vi "Create Folders.vi"(8 "error in (no error)":errorcluster, 11 "PostBuildSupport in":refnum<class "PostBuildSupport.lvclass">) -> (0 "error out":errorcluster, 3 "PostBuildSupport out":refnum<class "PostBuildSupport.lvclass">)   [LabVIEW 2016, in "PostBuildSupport.lvclass"]
uses:
  PostBuildSupport.lvclass
  PostBuildSupport.lvclass/PostBuildSupport.ctl
  <userlib>/_MGI/File/MGI Create Directory Chain Behavior Enum.ctl
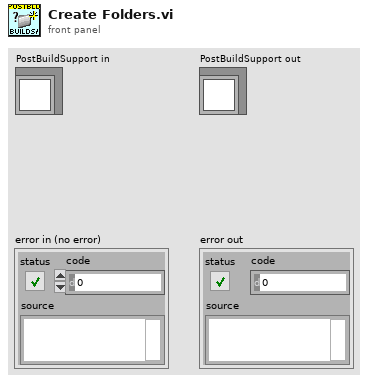
[diagram p1: front panel]
types:
  T1 = typedef "MGI Create Directory Chain Behavior Enum.ctl" = enum16{"Auto Detect", "Path Contains a File", "Path Does Not Contain a File"}
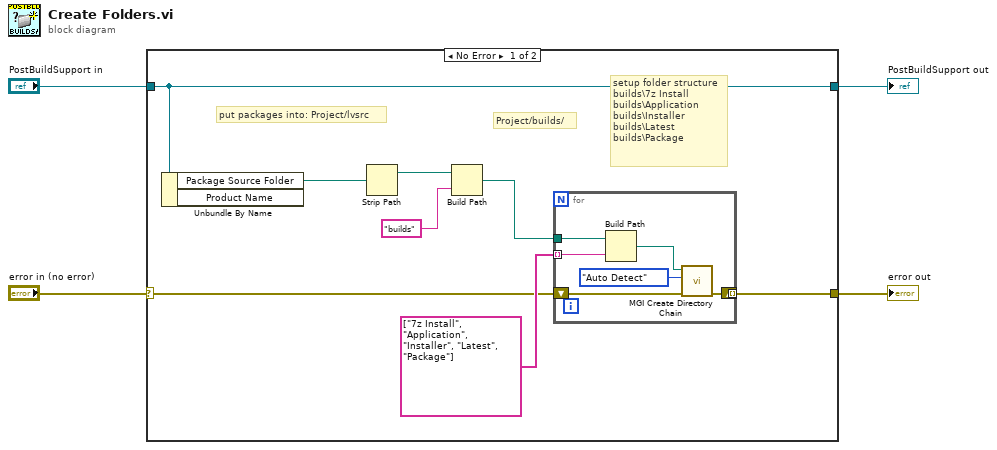
[diagram p0: block diagram]
diagram:
  n1 = case shown="No Error" "error in (no error)" {
    selector: "error in (no error)" -> [w9 w19]
    tunnel: "PostBuildSupport in" -> [w8 w20]
    tunnel: [w10 w19] -> w3
    tunnel: [w8 w20] -> w1
    frame No Error {
      # "Project/builds/"
      # "put packages into: Project/lvsrc"
      # "setup folder structure\nbuilds\\7z Install\nbuilds\\Application\nbuilds\\Installer\nbuilds\\Latest\nbuilds\\Package"
      n2 = Unbundle By Name(w8) -> ("Package Source Folder"=w11:path)  [unwired: 1 out]
      n3 = Strip Path(path=w11) -> (stripped path=w7:path)  [unwired: 1 out]
      n4 = Build Path(base path=w7, name or relative path="builds") -> (appended path=w5:path)
      n5 = for {
        shift-right: [w13] -> w10
        shift-left: w9 -> [w17]
        tunnel: w5 -> [w16]
        tunnel: string[] ["7z Install", "Application", "Installer", "Latest", "Package"] -> [w15] mode=indexing
        tunnel: [w13] -> _ mode=indexing
        n6 = Build Path(base path=w16, name or relative path=w15) -> (appended path=w14:path)
        n7 = call <userlib>:"MGI Create Directory Chain.vi"("Error In"=w17, "File Presence (Auto Detect)"=MGI_Create_Directory_Chain_Behavior_Enum."Auto Detect", "Path"=w14) -> ("Error Out"=w13:errorcluster)  [unwired: 7 in, 1 out]
      }
    }
    frame Error {
    }
  }
  "error out" <- w3
  "PostBuildSupport out" <- w1
